vi "Create Thread Pool.vi"(7 "number of threads":u16, 8 "error in (no error)":errorcluster, 10 "Thread type":refnum<class "Thread.lvclass">, 11 "Thread Pool type":refnum<class "Thread Pool.lvclass">) -> (0 "error out":errorcluster, 3 "Thread Pool out":refnum<class "Thread Pool.lvclass">)   [LabVIEW 2017, in "DSF Core.lvlib" / "Thread Pool.lvclass"]
uses:
  Thread Pool.lvclass
  Thread/Thread.lvclass
  Thread Pool.lvclass/Thread Pool.ctl
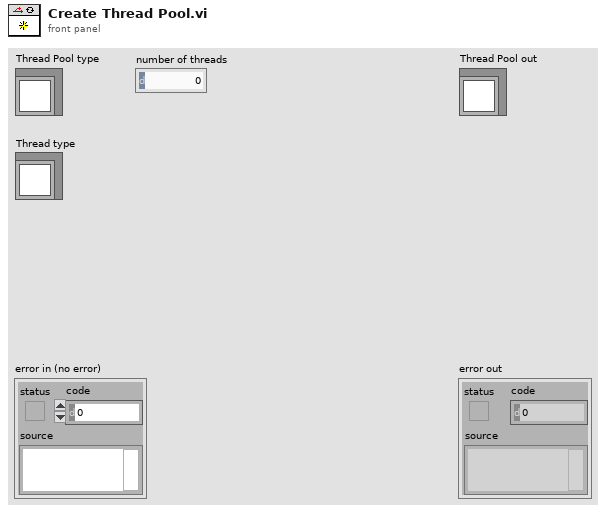
[diagram p1: front panel]
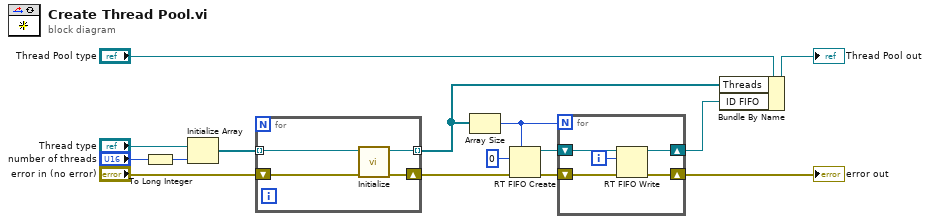
[diagram p0: block diagram]
diagram:
  n1 = To Long Integer(number="number of threads") -> (32bit integer=w13:i32)
  n2 = Initialize Array("Thread type", w13) -> (w12:refnum<class "Thread.lvclass">[])
  n3 = for {
    tunnel: w12 -> [w19] mode=indexing
    tunnel: [w18] -> w3 mode=indexing
    shift-right: [w17] -> w6
    shift-left: "error in (no error)" -> [w16]
    n4 = call-dynamic "Initialize.vi"("error in (no error)"=w16, "Thread in"=w19) -> ("error out"=w17:errorcluster, "Thread out"=w18:refnum<class "Thread.lvclass">)  [unwired: 8 in]
  }
  n5 = Array Size(array=w3) -> (size(s)=w1:i32)
  n6 = RT FIFO Create(1:0, 3:w6, 4:w1) -> (8:w4:refnum<k33>, 11:w5:errorcluster)  [unwired: 5 in, 1 out]
  n7 = for {
    N: w1 -> [_]
    shift-right: [w20] -> w8
    shift-left: w5 -> [w23]
    shift-right: [w21] -> w2
    shift-left: w4 -> [w24]
    i -> [w22]
    n8 = RT FIFO Write(0:w24, 1:w22, 3:w23) -> (8:w21:refnum<k33>, 11:w20:errorcluster)  [unwired: 2 in, 2 out]
  }
  "error out" <- w8
  n9 = Bundle By Name(cluster="Thread Pool type", "Threads"=w3, "ID FIFO"=w2) -> (→"Thread Pool out":refnum<class "Thread Pool.lvclass">)
